vi "define.vi"(8 "error in (no error)":errorcluster, 11 "TrajectoryCN090716SpiralScan in":refnum<class "TrajectoryCN090716SpiralScan.lvclass">) -> (0 "error out":errorcluster, 3 "TrajectoryCN090716SpiralScan out":refnum<class "TrajectoryCN090716SpiralScan.lvclass">)   [LabVIEW 2010, in "TrajectoryCN090716SpiralScan.lvclass"]
uses:
  TrajectoryCN090716SpiralScan.lvclass
  common/xcontrols/XImage/XImage/XImage.xctl
  common/classes/ImageCollection/ImageCollection/ImageCollection.lvclass
  common/xcontrols/XIntensityCompensation/XIntensityCompensation/XIntensityCompensation.xctl
  <vilib>/Math Plots/3D Math Plots/3D Scatter/3D Scatter XCtrl/3D Scatter.xctl
  common/xcontrols/XImage/XImage/ROI_mode_enum.ctl
  TrajectoryCN090716SpiralScan.lvclass/TrajectoryCN090716SpiralScan.ctl
  common/classes/ImageCollection/ImageCollection/add_mode_enum.ctl
  common/classes/Image/Image/Image.lvclass
  common/enumerations/functional_global_action_enum.ctl
  common/enumerations/x_y_z_enumeration.ctl
  <vilib>/Math Plots/3D Math Plots/3D Scatter/3D Scatter Datatype/Public/Plot Helper (Vector).vi
  <vilib>/Math Plots/3D Math Plots/3D Scatter/3D Scatter Datatype/3D Scatter Datatype.lvclass
panel:
  out "total number of pixels per cycle":i32
  in  "repetition rate":dbl[unit]
  in  "phase delay":dbl[unit]
  in  "correction factor":dbl
  out "parameters ok?":bool
  in  "Tab Control":T1(tab)
  in  "XImage":refnum<class "ImageCollection.lvclass">(xcontrol)
  in  "Intensity compensation":cluster{"depth":dbl[unit], "intensity":dbl}[](xcontrol)
  out "3D Scatter":refnum<class "3D Plot Datatype.lvclass">[](xcontrol)
  in  "cancel":bool
  in  "ok":bool
  in  "z amplitude":dbl[unit](slide)
  in  "spiral amplitude":dbl[unit](slide) min=0.0
  in  "spirals":i32(slide) scale=0.0..10.0
  in  "pixels  per turn":i32(slide) min=10 max=500 scale=10.0..500.0
  in  "turns":i32(slide) scale=1.0..30.0
  in  "z motion":enum16{"Sine", "Saw-tooth"}(ring)
  in  "circularity":dbl(slide) scale=0.0..1.0
  # "Define trajectory"
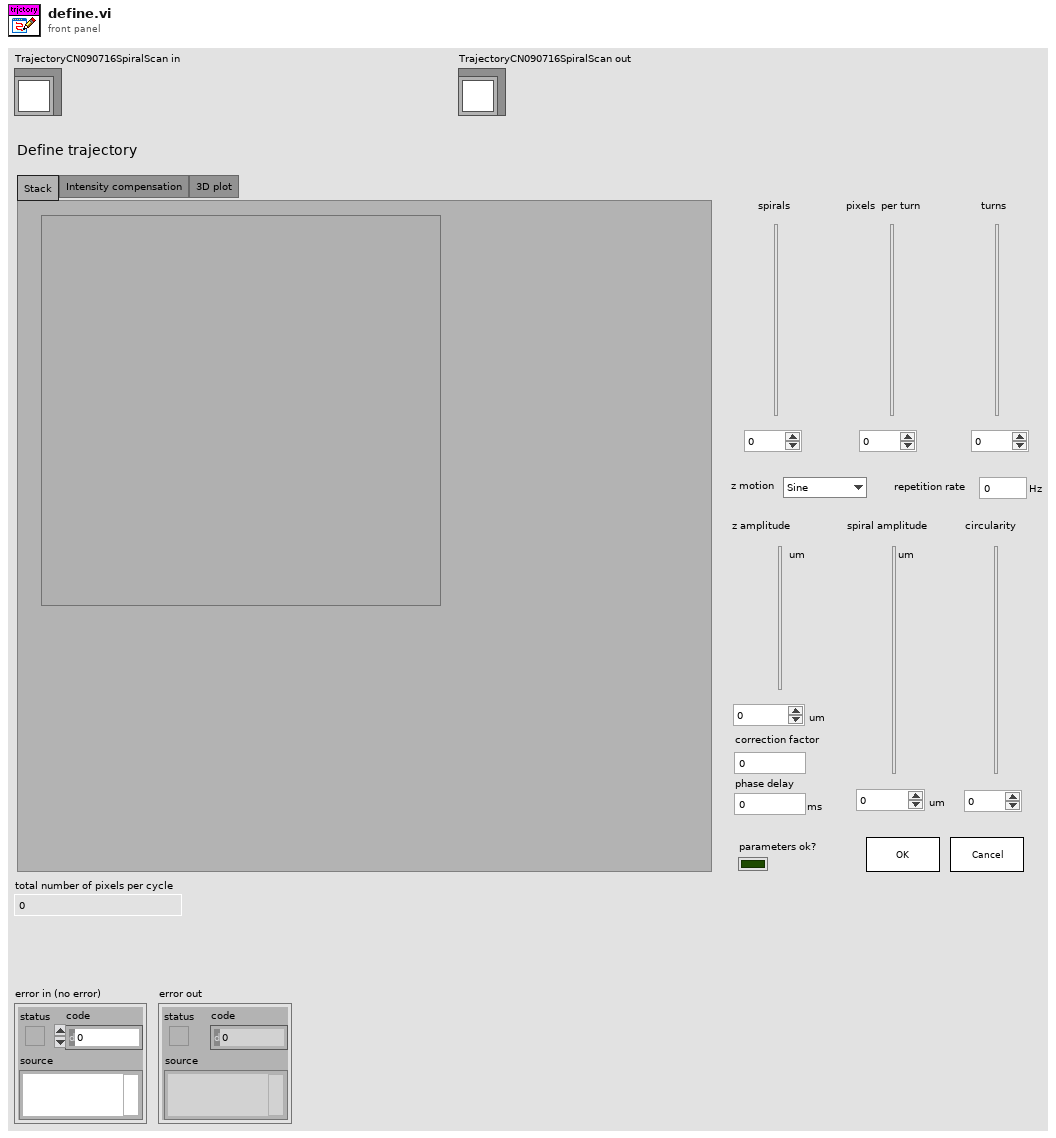
[diagram p1: front panel]
types:
  T1 = enum32{"Stack", "Intensity compensation", "3D plot"}
  T2 = typedef "XImage.xctl/ROI_mode_enum.ctl" = enum16{"none", "IMAQROIs", "PointCollection"}
  T3 = typedef "ImageCollection.lvclass/add_mode_enum.ctl" = enum16{"instance", "copy"}
  T4 = typedef "functional_global_action_enum.ctl" = enum16{"get", "set", "reset"}
  T5 = typedef "x_y_z_enumeration.ctl" = enum16{"x", "y", "z"}
  T6 = typedef "XImage.xctl/last_action_enum.ctl" = enum16{"not specified", "image loaded", "frame changed", "ROIs changed"}
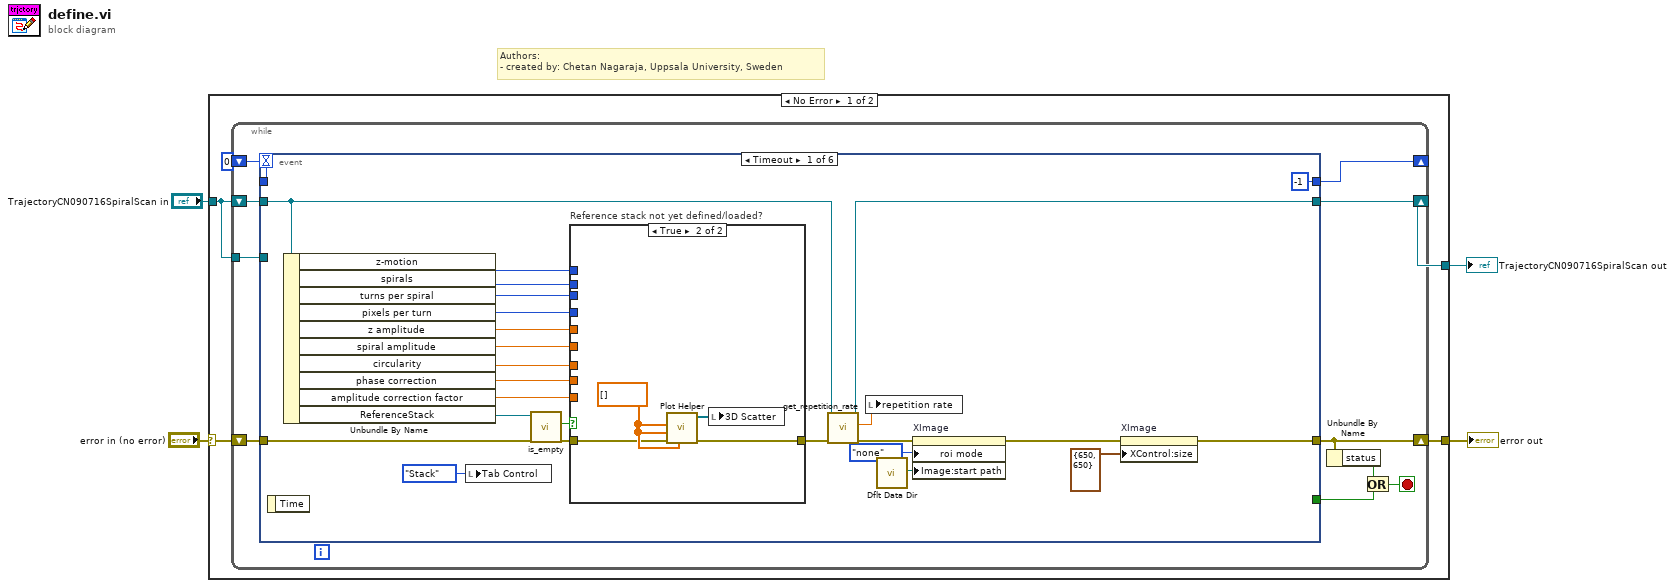
[diagram p0: block diagram]
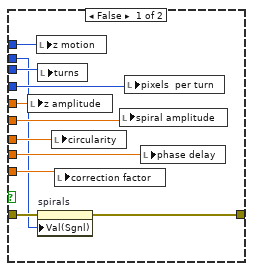
[diagram p2: hidden frame]
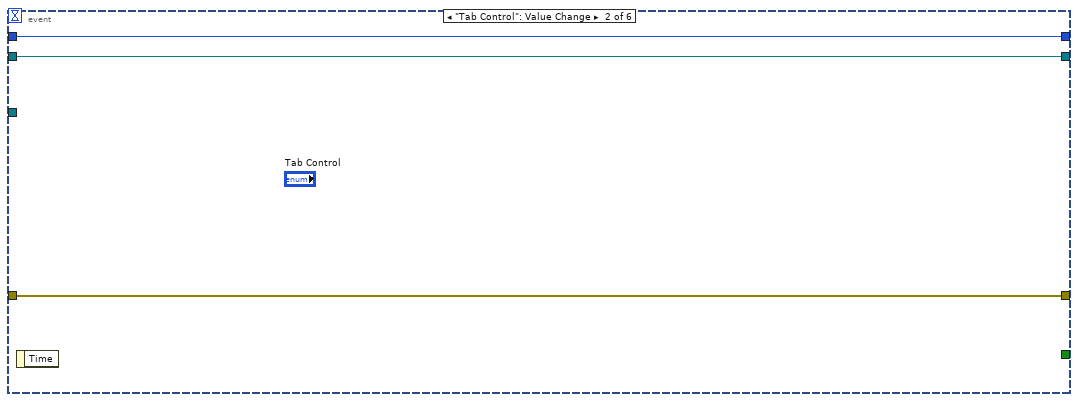
[diagram p3: hidden frame]
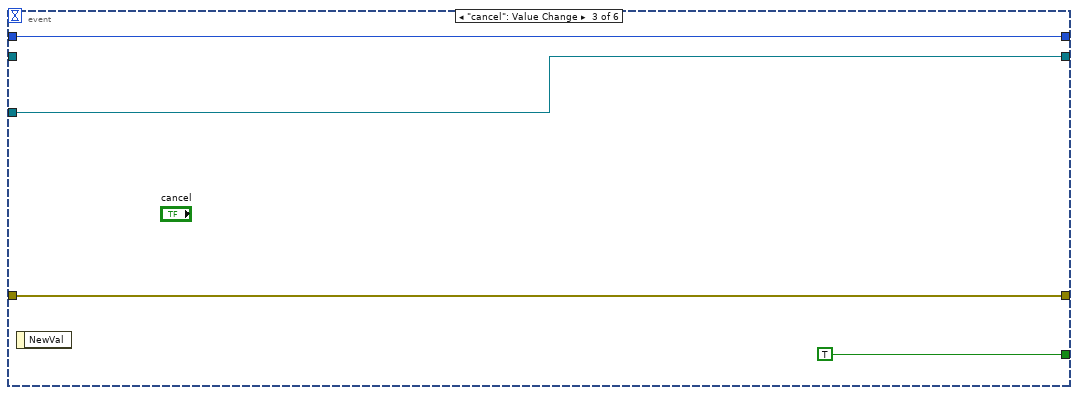
[diagram p4: hidden frame]
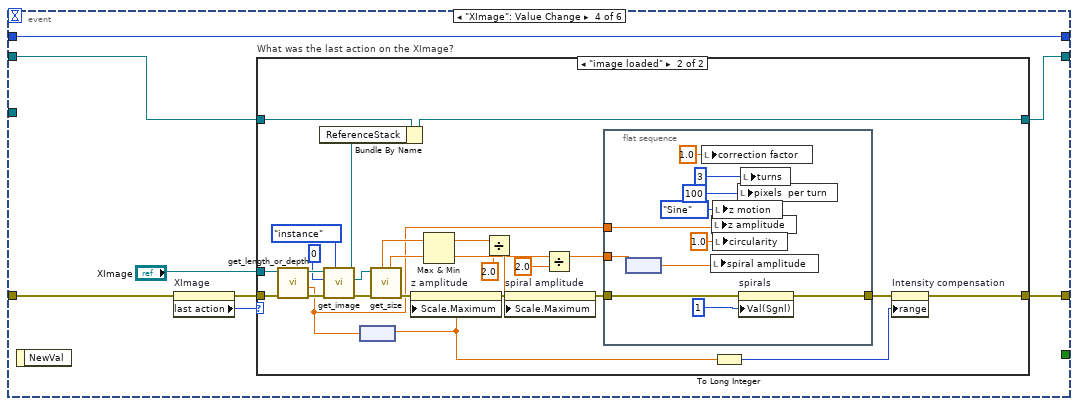
[diagram p5: hidden frame]
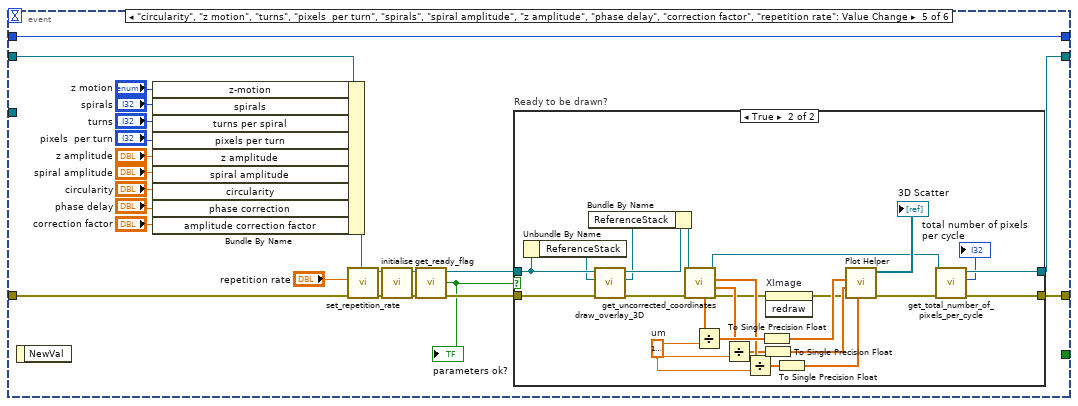
[diagram p7: hidden frame]
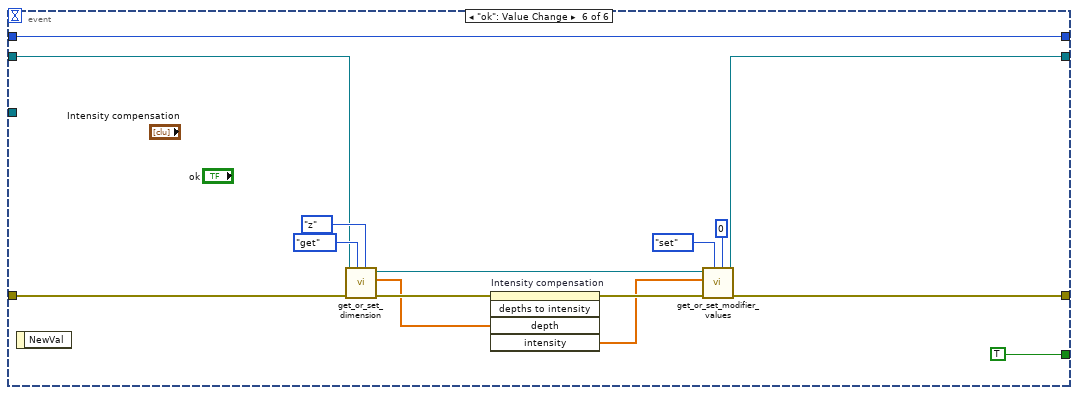
[diagram p9: hidden frame]
diagram:
  # "Authors: \n- created by: Chetan Nagaraja, Uppsala University, Sweden"
  n1 = case shown="No Error" "error in (no error)" {
    selector: "error in (no error)" -> [w9 w181]
    tunnel: [w7 w181] -> w3
    tunnel: [w8 w180] -> w1
    tunnel: "TrajectoryCN090716SpiralScan in" -> [w6 w180]
    frame No Error {
      n2 = while {
        shift-right: [w16] -> w7
        shift-left: w9 -> [w19]
        shift-right: [w17] -> w8
        shift-left: w6 -> [w18]
        tunnel: w6 -> [w12]
        shift-right: [w11] -> _
        shift-left: 0 -> [w10]
        stop <- w13 stop-if-true
        n3 = event shown="[0] Timeout" {
          selector: _ -> [_ _ _ _ _ _]
          dyn-events: _ -> [_ _ _ _ _ _]
          timeout: w10 -> [_ _ _ _ _ _]
          tunnel: w19 -> [w43 w62 w66 w69 w119 w176]
          tunnel: [w21 w62 w66 w71 w137 w170] -> w16
          tunnel: [_ _ TRUE _ _ TRUE] -> w14
          tunnel: w18 -> [w25 w60 _ w74 w129 w167]
          tunnel: [w24 w60 w64 w73 w136 w165] -> w17
          tunnel: w12 -> [_ _ w64 _ _ _]
          tunnel: w10 -> [_ w61 w63 w72 w135 w179]
          tunnel: [-1 w61 w63 w72 w135 w179] -> w11
          event Timeout {
            n4 = event-data() -> ()  [unwired: 1 in, 1 out]
            n5 = Unbundle By Name(w25) -> ("z-motion"=w31:enum16{"Sine", "Saw-tooth"}, "spirals"=w30:i32, "turns per spiral"=w32:i32, "pixels per turn"=w33:i32, "z amplitude"=w34:dbl[unit], "spiral amplitude"=w35:dbl[unit], "circularity"=w36:dbl, "phase correction"=w37:dbl[unit], "amplitude correction factor"=w38:dbl, "ReferenceStack"=w39:refnum<class "ImageCollection.lvclass">)
            n6 = local write "Tab Control"(T1."Stack" ("Tab Control")) -> ()
            n7 = call "is_empty.vi"("error in (no error)"=w43, "ImageCollection in"=w39) -> ("error out"=w42:errorcluster, "is empty?"=w41:bool)  [unwired: 7 in, 1 out]
            n8 = case "Reference stack not yet defined/loaded?" shown="True" w41 {
              tunnel: [w54 w56] -> w28
              tunnel: w42 -> [w55 w57]
              tunnel: w38 -> [w53 _]
              tunnel: w37 -> [w52 _]
              tunnel: w36 -> [w51 _]
              tunnel: w35 -> [w50 _]
              tunnel: w34 -> [w49 _]
              tunnel: w33 -> [w48 _]
              tunnel: w32 -> [w47 _]
              tunnel: w31 -> [w46 _]
              tunnel: w30 -> [w45 _]
              frame False {
                n9 = local write "z amplitude"(w49) -> ()
                n10 = local write "z motion"(w46) -> ()
                n11 = local write "turns"(w47) -> ()
                n12 = property on="spirals" class="Slide (strict)"(error in=w55, "Val(Sgnl)"=w45) -> (error out=w54:errorcluster)  [unwired: 1 in, 1 out]
                n13 = local write "circularity"(w51) -> ()
                n14 = local write "correction factor"(w53) -> ()
                n15 = local write "spiral amplitude"(w50) -> ()
                n16 = local write "pixels  per turn"(w48) -> ()
                n17 = local write "phase delay"(w52) -> ()
              }
              frame True {
                w59 = sgl[] [] ("x vector")
                n18 = call-poly <vilib>:"Plot Helper.vi"("z vector"=w59, "error in (no error)"=w57, "y vector"=w59, "x vector"=w59) -> ("error out"=w56:errorcluster, "3D Plot lvclass Array out"=w58:refnum<class "3D Plot Datatype.lvclass">[])  [unwired: 2 in, 4 out]
                n19 = local write "3D Scatter"(w58) -> ()
              }
            }
            n20 = call-dynamic "get_repetition_rate.vi"("error in (no error)"=w28, "GenericTrajectory in"=w25) -> ("error out"=w27:errorcluster, "repetition rate"=w26:dbl[unit], "GenericTrajectory out"=w24:refnum<class "TrajectoryCN090716SpiralScan.lvclass">)  [unwired: 7 in]
            n21 = local write "repetition rate"(w26) -> ()
            n22 = call <vilib>:"Dflt Data Dir.vi"() -> ("App:Default Data Directory"=w40:path)
            n23 = property on="XImage" class="XImage (strict)"(error in=w27, "roi mode"=ROI_mode_enum."none" ("ROI:mode"), "Image:start path"=w40) -> (error out=w22:errorcluster)  [unwired: 1 in, 1 out]
            n24 = property on="XImage" class="XImage (strict)"(error in=w22, "XControl:size"=cluster{"Width":u32, "Height":u32} {"Width"=650, "Height"=650}) -> (error out=w21:errorcluster)  [unwired: 1 in, 1 out]
          }
          event "Tab Control": Value Change {
            n25 = event-data() -> ()  [unwired: 1 in, 1 out]
          }
          event "cancel": Value Change {
            n26 = event-data() -> ()  [unwired: 1 in, 1 out]
          }
          event "XImage": Value Change {
            n27 = event-data() -> ()  [unwired: 1 in, 1 out]
            n28 = property on="XImage" class="XImage (strict)"(error in=w69) -> (error out=w68:errorcluster, "last action"=w67:T6)  [unwired: 1 in, 1 out]
            n29 = case "What was the last action on the XImage?" shown="\"image loaded\"" w67 {
              tunnel: w74 -> [w76 w103]
              tunnel: [w76 w102] -> w73
              tunnel: [w75 w81] -> w71
              tunnel: "XImage" -> [_ w94]
              tunnel: w68 -> [w75 w90]
              frame Default {
              }
              frame "image loaded" {
                n30 = call "get_length_or_depth.vi"("error in (no error)"=w90, "ImageCollection in"=w94) -> ("error out"=w99:errorcluster, "total z depth"=w78:dbl[unit], "ImageCollection out"=w101:refnum<class "ImageCollection.lvclass">)  [unwired: 5 in, 2 out]
                n31 = call-dynamic "get_image.vi"("get image as..."=add_mode_enum."instance", "error in (no error)"=w99, "index"=0, "ImageCollection in"=w101) -> ("error out"=w98:errorcluster, "Image.lvclass"=w97:refnum<class "Image.lvclass">, "ImageCollection out"=w100:refnum<class "ImageCollection.lvclass">)  [unwired: 5 in]
                n32 = Bundle By Name(cluster=w103, "ReferenceStack"=w100) -> (w102:refnum<class "TrajectoryCN090716SpiralScan.lvclass">)
                n33 = node(w78) -> (w77:dbl)
                n34 = call-dynamic "get_size.vi"("error in (no error)"=w98, "Image in"=w97) -> ("error out"=w93:errorcluster, "physical size y"=w91:dbl, "physical size x"=w92:dbl)  [unwired: 2 in, 5 out]
                n35 = property on="z amplitude" class="Slide (strict)"(error in=w93, "Scale.Maximum"=w77) -> (error out=w89:errorcluster)  [unwired: 1 in, 1 out]
                n36 = Max & Min(x=w92, y=w91) -> (max(x,y)=w86:dbl, min(x,y)=w85:dbl)
                n37 = Divide(x=w86, y=2.0) -> (x/y=w87:dbl)
                n38 = property on="spiral amplitude" class="Slide (strict)"(error in=w89, "Scale.Maximum"=w87) -> (error out=w88:errorcluster)  [unwired: 1 in, 1 out]
                n39 = Divide(x=w85, y=2.0) -> (x/y=w84:dbl)
                n40 = flat-sequence {
                  tunnel: w88 -> [w114]
                  tunnel: [w113] -> w80
                  tunnel: w84 -> [w105]
                  tunnel: w78 -> [w108]
                  frame #0 {
                    n41 = node(w105) -> (w106:dbl[unit])
                    n42 = local write "correction factor"(1.0 ("correction factor")) -> ()
                    n43 = local write "spiral amplitude"(w106) -> ()
                    n44 = local write "z amplitude"(w108) -> ()
                    n45 = local write "z motion"(enum16{"Sine", "Saw-tooth"}."Sine" ("z motion")) -> ()
                    n46 = local write "circularity"(1.0 ("circularity")) -> ()
                    n47 = local write "pixels  per turn"(100 ("number of turns")) -> ()
                    n48 = property on="spirals" class="Slide (strict)"(error in=w114, "Val(Sgnl)"=1 ("Value (Signaling)")) -> (error out=w113:errorcluster)  [unwired: 1 in, 1 out]
                    n49 = local write "turns"(3 ("number of turns")) -> ()
                  }
                }
                n50 = To Long Integer(number=w77) -> (32bit integer=w79:i32)
                n51 = property on="Intensity compensation" class="XIntensityCompensation (strict)"(error in=w80, "range"=w79) -> (error out=w81:errorcluster)  [unwired: 1 in, 1 out]
              }
            }
          }
          event "circularity", "z motion", "turns", "pixels  per turn", "spirals", "spiral amplitude", "z amplitude", "phase delay", "correction factor", "repetition rate": Value Change {
            n52 = event-data() -> ()  [unwired: 1 in, 1 out]
            n53 = Bundle By Name(cluster=w129, "z-motion"="z motion", "spirals"="spirals", "turns per spiral"="turns", "pixels per turn"="pixels  per turn", "z amplitude"="z amplitude", "spiral amplitude"="spiral amplitude", "circularity"="circularity", "phase correction"="phase delay", "amplitude correction factor"="correction factor") -> (w117:refnum<class "TrajectoryCN090716SpiralScan.lvclass">)
            n54 = call-dynamic "set_repetition_rate.vi"("error in (no error)"=w119, "repetition rate"="repetition rate", "GenericTrajectory in"=w117) -> ("error out"=w118:errorcluster, "GenericTrajectory out"=w116:refnum<class "TrajectoryCN090716SpiralScan.lvclass">)  [unwired: 7 in]
            n55 = call-dynamic "initialise.vi"("error in (no error)"=w118, "TrajectoryCN090716SpiralScan in"=w116) -> ("error out"=w133:errorcluster, "TrajectoryCN090716SpiralScan out"=w134:refnum<class "TrajectoryCN090716SpiralScan.lvclass">)  [unwired: 8 in]
            n56 = call-dynamic "get_ready_flag.vi"("error in (no error)"=w133, "GenericTrajectory in"=w134) -> ("error out"=w132:errorcluster, "ready for initialisation?"=w130:bool, "GenericTrajectory out"=w131:refnum<class "TrajectoryCN090716SpiralScan.lvclass">)  [unwired: 7 in]
            "parameters ok?" <- w130
            n57 = case "Ready to be drawn?" shown="True" w130 {
              tunnel: [w139 w156] -> w137
              tunnel: [w138 w155] -> w136
              tunnel: w131 -> [w138 w164]
              tunnel: w132 -> [w139 w163]
              frame False {
              }
              frame True {
                w157 = dbl[unit] 1e-06  # um
                n58 = Unbundle By Name(w164) -> ("ReferenceStack"=w162:refnum<class "ImageCollection.lvclass">)
                n59 = call-dynamic "draw_overlay_3D.vi"("error in (no error)"=w163, "ImageCollection in"=w162, "GenericTrajectory in"=w164) -> ("error out"=w159:errorcluster, "ImageCollection out"=w160:refnum<class "ImageCollection.lvclass">, "GenericTrajectory out"=w161:refnum<class "TrajectoryCN090716SpiralScan.lvclass">)  [unwired: 6 in]
                n60 = Bundle By Name(cluster=w161, "ReferenceStack"=w160) -> (w158:refnum<class "TrajectoryCN090716SpiralScan.lvclass">)
                n61 = call-dynamic "get_uncorrected_coordinates.vi"("error in (no error)"=w159, "TrajectoryCN090716SpiralScan in"=w158) -> ("error out"=w142:errorcluster, "y"=w150:dbl[unit][], "z"=w149:dbl[unit][], "TrajectoryCN090716SpiralScan out"=w146:refnum<class "TrajectoryCN090716SpiralScan.lvclass">, "x"=w151:dbl[unit][])  [unwired: 5 in]
                n62 = Divide(x=w151, y=w157) -> (x/y=w152:dbl[])
                n63 = Divide(x=w150, y=w157) -> (x/y=w148:dbl[])
                n64 = Divide(x=w149, y=w157) -> (x/y=w147:dbl[])
                n65 = To Single Precision Float(number=w152) -> (single precision float=w143:sgl[])
                n66 = To Single Precision Float(number=w148) -> (single precision float=w144:sgl[])
                n67 = invoke on="XImage" class="XImage (strict)" method="redraw"(error in=w142) -> (error out=w141:errorcluster)  [unwired: 2 in, 2 out]
                n68 = To Single Precision Float(number=w147) -> (single precision float=w145:sgl[])
                n69 = call-poly <vilib>:"Plot Helper.vi"("z vector"=w145, "error in (no error)"=w141, "y vector"=w144, "x vector"=w143) -> ("error out"=w140:errorcluster, "3D Plot lvclass Array out"=→"3D Scatter":refnum<class "3D Plot Datatype.lvclass">[])  [unwired: 2 in, 4 out]
                n70 = call-dynamic "get_total_number_of_pixels_per_cycle.vi"("error in (no error)"=w140, "GenericTrajectory in"=w146) -> ("error out"=w156:errorcluster, "total number of pixels per cycle"=→"total number of pixels per cycle":i32, "GenericTrajectory out"=w155:refnum<class "TrajectoryCN090716SpiralScan.lvclass">)  [unwired: 7 in]
              }
            }
          }
          event "ok": Value Change {
            n71 = event-data() -> ()  [unwired: 1 in, 1 out]
            n72 = call-dynamic "get_or_set_dimension.vi"("dimension"=x_y_z_enumeration."z", "action"=functional_global_action_enum."get", "error in (no error)"=w176, "GenericTrajectory in"=w167) -> ("error out"=w174:errorcluster, "pixel values out (single dimension)"=w169:dbl[unit][], "GenericTrajectory out"=w166:refnum<class "TrajectoryCN090716SpiralScan.lvclass">)  [unwired: 5 in]
            n73 = invoke on="Intensity compensation" class="XIntensityCompensation (strict)" method="depths to intensity"(error in=w174, "depth"=w169) -> (error out=w171:errorcluster, "intensity"=w168:dbl[])  [unwired: 3 in, 3 out]
            n74 = call-dynamic "get_or_set_modifier_values.vi"("modifier index"=0, "action"=functional_global_action_enum."set", "error in (no error)"=w171, "modifier values in"=w168, "GenericTrajectory in"=w166) -> ("error out"=w170:errorcluster, "GenericTrajectory out"=w165:refnum<class "TrajectoryCN090716SpiralScan.lvclass">)  [unwired: 4 in, 1 out]
          }
        }
        n75 = Unbundle By Name(w16) -> ("status"=w15:bool)
        n76 = Or(x=w15, y=w14) -> (x .or. y?=w13:bool)
      }
    }
    frame Error {
    }
  }
  "error out" <- w3
  "TrajectoryCN090716SpiralScan out" <- w1
